vi "Digitizer DC Voltage Configure.vi"(0 "instrument handle":refnum<k15>, 1 "Mode (Time)":i32(ring) items=["Time", "Frequency"], 2 "SampRate":dbl format="%#_6f", 5 "Range":dbl format="%#_6f", 7 "InputType (Differential)":i32(ring) items=["Differential", "Sended"], 9 "Coupling (DC)":i32(ring) items=["DC", "AC"], 11 "error in (no error)":errorcluster {"code" format="%.0x"}, 12 "SampCount":i32, 13 "ChannelList":string) -> (4 "instrument handle out":refnum<k15>, 15 "error out":errorcluster {"code" format="%.0x"})   [LabVIEW 2020, in "Keysight DAQ970.lvlib"]
doc: "Configures the channels for DC voltage module digitizing, but they do not initiate the digitizing."
uses:
  Keysight DAQ970.lvlib
  KtDAQ970.dll
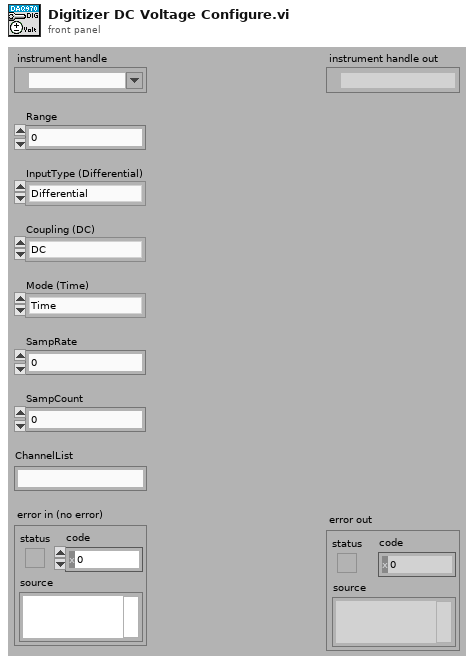
[diagram p1: front panel]
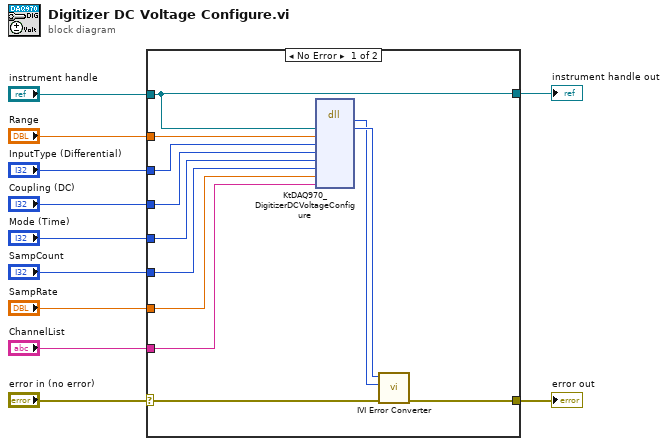
[diagram p0: block diagram]
diagram:
  n1 = case shown="No Error" "error in (no error)" {
    selector: "error in (no error)" -> [w21 w25]
    tunnel: [w20 w25] -> w11
    tunnel: "instrument handle" -> [w12 w24]
    tunnel: "Range" -> [w19 _]
    tunnel: "InputType (Differential)" -> [w18 _]
    tunnel: "Coupling (DC)" -> [w17 _]
    tunnel: "Mode (Time)" -> [w16 _]
    tunnel: "SampCount" -> [w15 _]
    tunnel: "SampRate" -> [w14 _]
    tunnel: "ChannelList" -> [w13 _]
    tunnel: [w12 w24] -> w1
    frame No Error {
      n2 = dll-call lib="KtDAQ970**.dll" fn="KtDAQ970_DigitizerDCVoltageConfigure"("Vi"=w12, "Range"=w19, "InputType"=w18, "Coupling"=w17, "Mode"=w16, "SampCount"=w15, "SampRate"=w14, "ChannelList"=w13) -> (w22:i32, "Vi"=w23:u32)  [unwired: 10 in, 2 out]
      n3 = call "IVI Error Converter.vi"("error in (no error)"=w21, "IVI error code (0)"=w22, "instrument handle"=w23) -> ("error out"=w20:errorcluster)  [unwired: 7 in, 1 out]
    }
    frame Error {
    }
  }
  "error out" <- w11
  "instrument handle out" <- w1
